vi "Create BIN list.vi"(9 "Bin Width":dbl, 10 "Min":dbl, 11 "Max":dbl) -> (3 "Bins":T1(array[cluster]) {"upper" format="%0.2f"; "lower" format="%0.2f"})   [LabVIEW 2011]
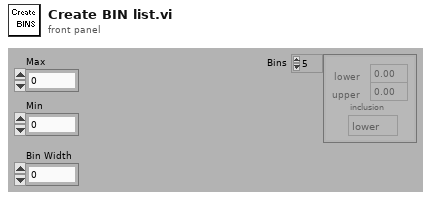
[diagram p1: front panel]
types:
  T1 = cluster{"lower":dbl, "upper":dbl, "inclusion":enum32{"lower", "upper", "both", "neither"}}[]
  T2 = cluster{"lower":dbl, "upper":dbl, "inclusion":enum32{"lower", "upper", "both", "neither"}}
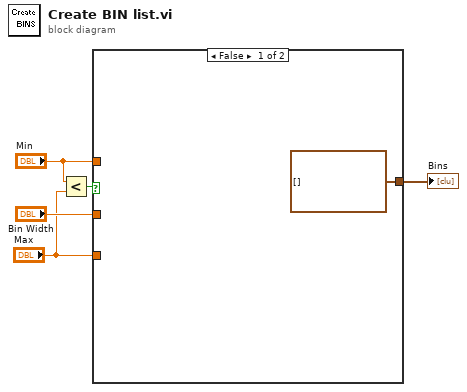
[diagram p0: block diagram]
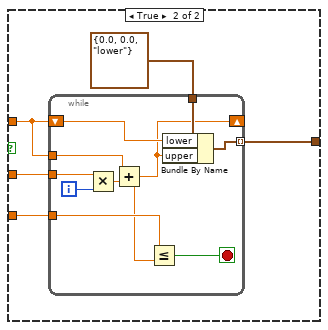
[diagram p2: hidden frame]
diagram:
  n1 = Less?(x="Min", y="Max") -> (x < y?=w1:bool)
  n2 = case shown="False" w1 {
    tunnel: [T1 [] w10] -> w5
    tunnel: "Bin Width" -> [_ w9]
    tunnel: "Min" -> [_ w8]
    tunnel: "Max" -> [_ w7]
    frame False {
    }
    frame True {
      n3 = while {
        tunnel: T2 {"lower"=0.0, "upper"=0.0, "inclusion"=enum."lower"} -> [w21]
        tunnel: [w20] -> w10 mode=indexing
        tunnel: w9 -> [w19]
        shift-right: [w13] -> _
        shift-left: w8 -> [w16]
        tunnel: w8 -> [w15]
        tunnel: w7 -> [w14]
        i -> [w18]
        stop <- w12 stop-if-true
        n4 = Multiply(x=w19, y=w18) -> (x*y=w17:dbl)
        n5 = Add(x=w15, y=w17) -> (x+y=w13:dbl)
        n6 = Less Or Equal?(x=w14, y=w13) -> (x <= y?=w12:bool)
        n7 = Bundle By Name(cluster=w21, "lower"=w16, "upper"=w13) -> (w20:T2)
      }
    }
  }
  "Bins" <- w5
